vi "branin.vi"(7 "LabVIEW Web Service Request":refnum<class "Web Request.lvclass">) -> (3 "result":dbl)   [LabVIEW 2019]
uses:
  <vilib>/wsapi/Web Request.lvclass
panel:
  out "indic":dbl[](array[numeric])
  out "processed":string[][](array[string])
  out "Constituents":i32
  out "Splits":i32
  out "postdata":string
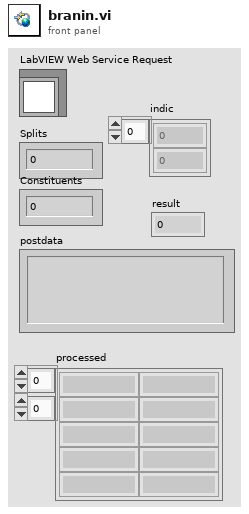
[diagram p1: front panel]
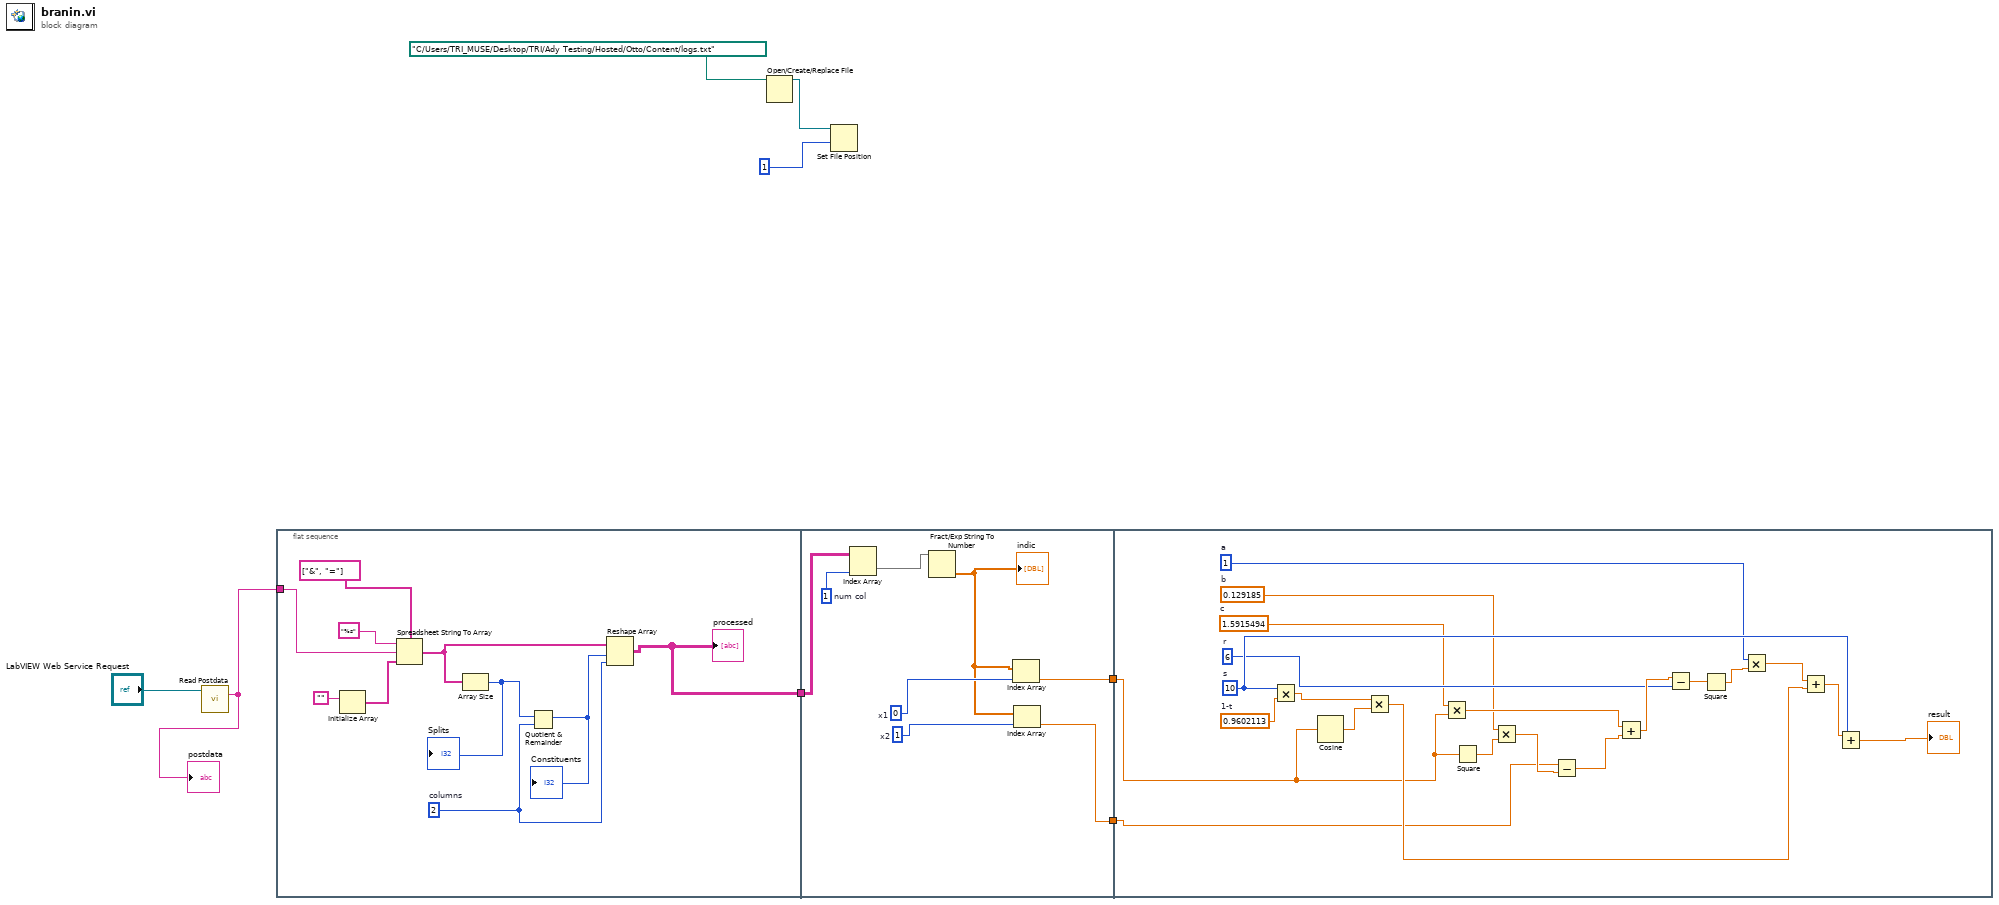
[diagram p0: block diagram]
diagram:
  n1 = call <vilib>:"Read Postdata.vi"("LabVIEW Web Service Request"="LabVIEW Web Service Request") -> ("postdata"=w4:string)  [unwired: 12 in, 2 out]
  "postdata" <- w4
  n2 = flat-sequence {
    tunnel: w4 -> [w9]
    tunnel: [w10] -> w8
    tunnel: w8 -> [w25]
    tunnel: [w22] -> w7
    tunnel: [w21] -> w6
    tunnel: w7 -> [w29]
    tunnel: w6 -> [w28]
    frame #0 {
      w13 = 2  # columns
      n3 = Initialize Array("") -> (w15:string[])  [unwired: 1 in]
      n4 = Spreadsheet String To Array(delimiter (Tab)=string[] ["&", "="], format string="%s", spreadsheet string=w9, array type (2D Dbl)=w15) -> (array=w11:string[])
      n5 = Array Size(array=w11) -> (size(s)=w14:i32)
      "Splits" <- w14
      n6 = Quotient & Remainder(x=w14, y=w13) -> (floor(x/y)=w12:i32)  [unwired: 1 out]
      "Constituents" <- w12
      n7 = Reshape Array(w11, w12, w13) -> (w10:string[][])
      "processed" <- w10
    }
    frame #1 {
      w24 = 0  # x1
      w23 = 1  # x2
      w26 = 1  # num col
      n8 = Index Array(array=w25, index (col)=w26) -> (element=w20:string[])  [unwired: 1 in]
      n9 = Fract/Exp String To Number(string=w20) -> (number=w19:dbl[])  [unwired: 3 in, 1 out]
      "indic" <- w19
      n10 = Index Array(array=w19, index=w24) -> (element=w22:dbl)
      n11 = Index Array(array=w19, index=w23) -> (element=w21:dbl)
    }
    frame #2 {
      w34 = 0.9602113  # 1-t
      w35 = 10  # s
      w32 = 6  # r
      w31 = 1.5915494  # c
      w30 = 0.129185  # b
      w33 = 1  # a
      n12 = Multiply(x=w35, y=w34) -> (x*y=w41:dbl)
      n13 = Cosine(x=w29) -> (cos(x)=w42:dbl)
      n14 = Multiply(x=w41, y=w42) -> (x*y=w44:dbl)
      n15 = Multiply(x=w31, y=w29) -> (x*y=w38:dbl)
      n16 = Square(x=w29) -> (x^2=w36:dbl)
      n17 = Multiply(x=w30, y=w36) -> (x*y=w37:dbl)
      n18 = Subtract(x=w28, y=w37) -> (x-y=w39:dbl)
      n19 = Add(x=w38, y=w39) -> (x+y=w40:dbl)
      n20 = Subtract(x=w40, y=w32) -> (x-y=w46:dbl)
      n21 = Square(x=w46) -> (x^2=w47:dbl)
      n22 = Multiply(x=w33, y=w47) -> (x*y=w43:dbl)
      n23 = Add(x=w43, y=w44) -> (x+y=w45:dbl)
      n24 = Add(x=w45, y=w35) -> (x+y=→"result":dbl)
    }
  }
  n25 = Open/Create/Replace File(file path (use dialog)=path "C:/Users/TRI_MUSE/Desktop/TRI/Ady Testing/Hosted/Otto/Content/logs.txt") -> (refnum out=w2:refnum<file>)  [unwired: 5 in, 2 out]
  n26 = Set File Position(refnum=w2, from (0:start)=1) -> ()  [unwired: 2 in, 2 out]
